vi "Copy Template Library.vi"(0 "configuration":T1, 11 "error in":errorcluster) -> (4 "project ref out":refnum<vi>, 15 "error out":errorcluster)   [LabVIEW 2021, in "InstrumentStudio Plug-In Editor.lvlib"]
uses:
  InstrumentStudio Plug-In Editor.lvlib
  controls/Data Holder.ctl
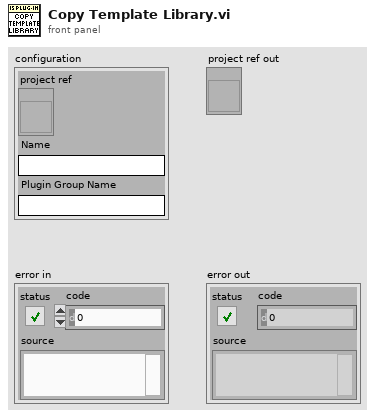
[diagram p1: front panel]
types:
  T1 = typedef "InstrumentStudio Plug-In Editor.lvlib/Data Holder.ctl" = cluster{"project ref":refnum<vi>, "Name":string, "Plugin Group Name":string}
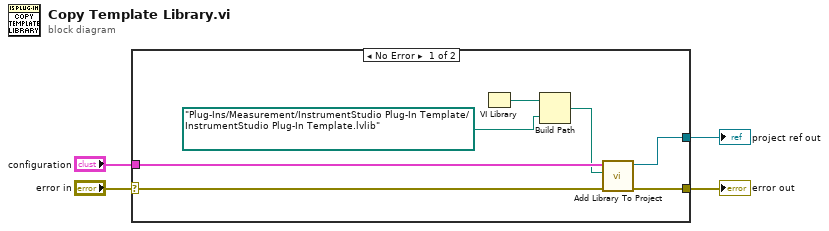
[diagram p0: block diagram]
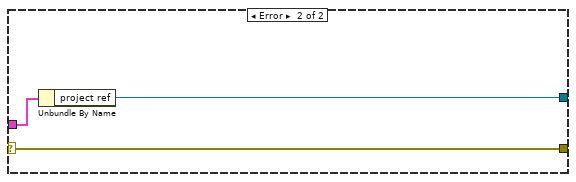
[diagram p2: hidden frame]
diagram:
  n1 = case shown="No Error" "error in" {
    selector: "error in" -> [w10 w14]
    tunnel: [w11 w14] -> w4
    tunnel: [w9 w12] -> w2
    tunnel: "configuration" -> [w8 w13]
    frame No Error {
      n2 = VI Library() -> (path=w7:path)
      n3 = Build Path(base path=w7, name or relative path=path "Plug-Ins/Measurement/InstrumentStudio Plug-In Template/InstrumentStudio Plug-In Template.lvlib") -> (appended path=w6:path)
      n4 = call "Add Library To Project.vi"("error in"=w10, "library path"=w6, "configuration"=w8) -> ("error out"=w11:errorcluster, "project ref out"=w9:refnum<vi>)  [unwired: 7 in]
    }
    frame Error {
      n5 = Unbundle By Name(w13) -> ("project ref"=w12:refnum<vi>)
    }
  }
  "error out" <- w4
  "project ref out" <- w2
